vi "Finalize.vi"(8 "error in (no error)":errorcluster) -> (0 "error out":errorcluster)   [LabVIEW 2014, in "lvprj2html.lvlib"]
uses:
  lvprj2html.lvlib
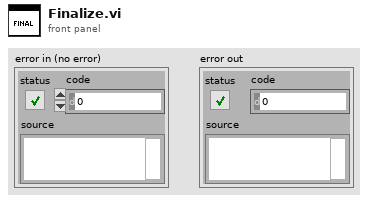
[diagram p1: front panel]
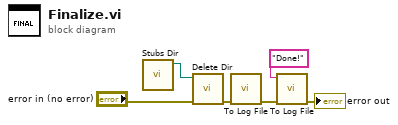
[diagram p0: block diagram]
diagram:
  n1 = call "Stubs Dir.vi"() -> ("path"=w4:path)  [unwired: 11 in]
  n2 = call "Delete Dir.vi"("error in (no error)"="error in (no error)", "dup path"=w4) -> ("error out"=w1:errorcluster)  [unwired: 8 in, 1 out]
  n3 = call "To Log File.vi"("error in (no error)"=w1) -> ("error out"=w2:errorcluster)  [unwired: 10 in]
  n4 = call "To Log File.vi"("error in (no error)"=w2, "string"="Done!" ("format string")) -> ("error out"=→"error out":errorcluster)  [unwired: 9 in]
